vi "Neighbors.vi"(5 "Position":T1, 7 "Board Size":i32, 11 "Team In":i32[][](array[numeric])) -> (2 "Neighbors":i32[](array[numeric]), 3 "Team":i32[][](array[numeric]))   [LabVIEW 2020, in "SquareBattle.lvlib" / "Map.lvclass"]
uses:
  Map.lvclass
  Position.ctl
  SquareBattle.lvlib
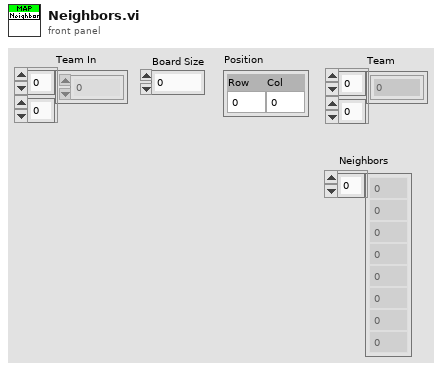
[diagram p1: front panel]
types:
  T1 = typedef "SquareBattle.lvlib/Position.ctl" = cluster{"Row":i32, "Col":i32}
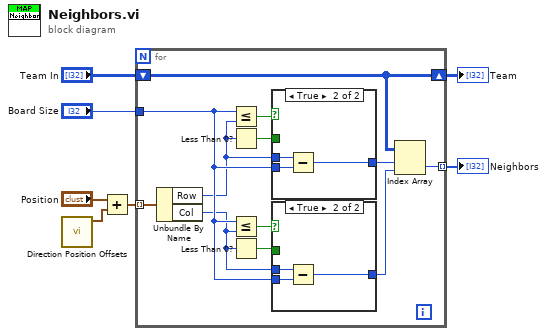
[diagram p0: block diagram]
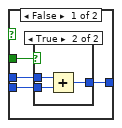
[diagram p2: hidden frame]
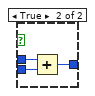
[diagram p5: hidden frame]
diagram:
  n1 = call "Direction Position Offsets.vi"() -> ("Direction Position Offsets"=w2:T1[])  [unwired: 11 in]
  n2 = Add(x="Position", y=w2) -> (x+y=w4:T1[])
  n3 = for {
    shift-right: [w19] -> w6
    shift-left: "Team In" -> [w19]
    tunnel: w4 -> [w16] mode=indexing
    tunnel: [w18] -> w3 mode=indexing
    tunnel: "Board Size" -> [w17]
    n4 = Unbundle By Name(w16) -> ("Row"=w11:i32, "Col"=w8:i32)
    n5 = Less Or Equal?(x=w17, y=w11) -> (x <= y?=w13:bool)
    n6 = Less Than 0?(x=w11) -> (x < 0?=w12:bool)
    n7 = Less Or Equal?(x=w17, y=w8) -> (x <= y?=w10:bool)
    n8 = Less Than 0?(x=w8) -> (x < 0?=w9:bool)
    n9 = case shown="True" w13 {
      tunnel: w12 -> [w34 _]
      tunnel: w11 -> [w33 w41]
      tunnel: w17 -> [w32 w40]
      tunnel: [w31 w39] -> w15
      frame False {
        n10 = case shown="False" w34 {
          tunnel: w33 -> [w35 w38]
          tunnel: w32 -> [_ w37]
          tunnel: [w35 w36] -> w31
          frame False {
          }
          frame True {
            n11 = Add(x=w38, y=w37) -> (x+y=w36:i32)
          }
        }
      }
      frame True {
        n12 = Subtract(x=w41, y=w40) -> (x-y=w39:i32)
      }
    }
    n13 = case shown="True" w10 {
      tunnel: w9 -> [w23 _]
      tunnel: w8 -> [w22 w30]
      tunnel: w17 -> [w21 w29]
      tunnel: [w20 w28] -> w14
      frame False {
        n14 = case shown="True" w23 {
          tunnel: w22 -> [w24 w27]
          tunnel: w21 -> [_ w26]
          tunnel: [w24 w25] -> w20
          frame False {
          }
          frame True {
            n15 = Add(x=w27, y=w26) -> (x+y=w25:i32)
          }
        }
      }
      frame True {
        n16 = Subtract(x=w30, y=w29) -> (x-y=w28:i32)
      }
    }
    n17 = Index Array(array=w19, index (row)=w15, index (col)=w14) -> (element=w18:i32)
  }
  "Team" <- w6
  "Neighbors" <- w3
